vi "Launcher.vi"   [LabVIEW 2020]
uses:
  User Interface/User Interface.lvclass
  C:/Program Files (x86)/National Instruments/LabVIEW 2020/vi.lib/ActorFramework/Actor/Actor.lvclass
  <vilib>/ActorFramework/Actor/Actor.lvclass
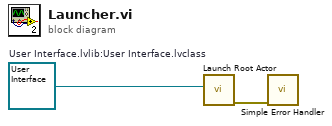
[diagram p0: block diagram]
diagram:
  w2 = refnum<class "User Interface.lvclass"> refnum  # User Interface.lvlib:User Interface.lvclass
  n1 = call <vilib>:"Launch Root Actor.vi"("Actor"=w2) -> ("error out"=w1:errorcluster)  [unwired: 9 in, 1 out]
  n2 = call <vilib>:"Simple Error Handler.vi"("error in (no error)"=w1) -> ()  [unwired: 4 in, 5 out]
